vi "Get Enable.vi"(8 "error in (no error)":errorcluster, 11 "Handle in":i32) -> (0 "error out":errorcluster, 2 "Enable?":bool, 3 "Handle out":i32)   [LabVIEW 2013, in "Thorlabs_MC2000B.lvlib"]
uses:
  <instrlib>/Thorlabs_MC2000B/Thorlabs_MC2000B.lvlib
  <instrlib>/Thorlabs_MC2000B/Library/MC2000CommandLibWin32.dll
  Program Files/National Instruments/LabVIEW 2011/instr.lib/Thorlabs_MC2000B/Library/MC2000CommandLibWin64.dll
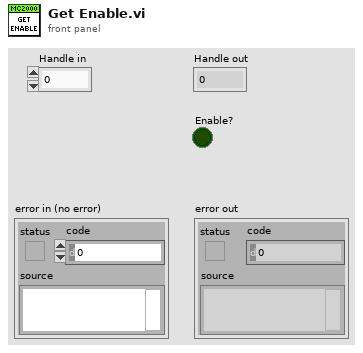
[diagram p1: front panel]
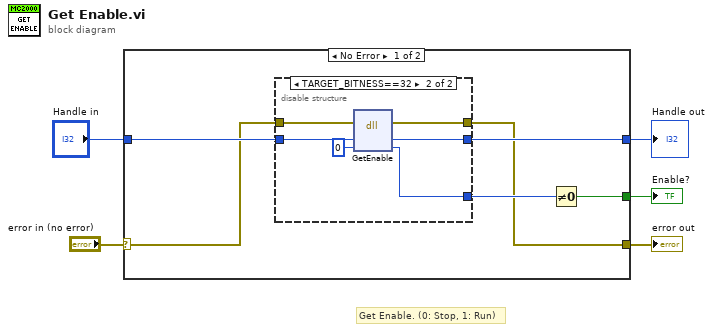
[diagram p0: block diagram]
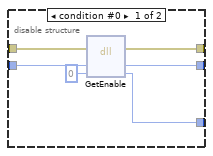
[diagram p2: hidden frame]
diagram:
  # "Get Enable. (0: Stop, 1: Run)"
  n1 = case shown="No Error" "error in (no error)" {
    selector: "error in (no error)" -> [w7 w25]
    tunnel: [w11 _] -> w5
    tunnel: [w6 w25] -> w4
    tunnel: "Handle in" -> [w10 w24]
    tunnel: [w9 w24] -> w1
    frame No Error {
      n2 = disable-structure shown="TARGET_BITNESS==32" {
        disable-tunnel: w10 -> [w17 w23]
        disable-tunnel: [w16 w22] -> w9
        disable-tunnel: [w15 w21] -> w8
        disable-tunnel: w7 -> [w13 w19]
        disable-tunnel: [w12 w18] -> w6
        frame condition #0 {
          n3 = dll-call lib="D:/Program Files/National Instruments/LabVIEW 2011/instr.lib/Thorlabs_MC2000B/Library/MC2000CommandLibWin64.dll" fn="GetEnable"(error in=w13, "hdl"=w17, "enable"=0) -> (error out=w12:errorcluster, "hdl"=w16:i32, "enable"=w15:i32)  [unwired: 3 in, 1 out]
        }
        frame condition #1 (active) {
          n4 = dll-call lib="C:/Program Files (x86)/National Instruments/LabVIEW 2013/instr.lib/Thorlabs_MC2000B/Library/MC2000CommandLibWin32.dll" fn="GetEnable"(error in=w19, "hdl"=w23, "enable"=0) -> (error out=w18:errorcluster, "hdl"=w22:i32, "enable"=w21:i32)  [unwired: 3 in, 1 out]
        }
      }
      n5 = Not Equal To 0?(x=w8) -> (x != 0?=w11:bool)
    }
    frame Error {
    }
  }
  "error out" <- w4
  "Enable?" <- w5
  "Handle out" <- w1
